vi "exnSpectralBlock spectral measurements peak array WFM.vi"(0 "Signals":waveform(dbl)[](graph), 5 "Restart Averaging":bool, 7 "View":T2, 9 "Spectrum Window":u16, 11 "error in (no error)":errorcluster, 12 "Spectrum Averaging Parameters":T1={"averaging mode"=0, "weighting mode"=1, "number of averages"=10} {"averaging mode" items=["No averaging", "Vector averaging", "RMS averaging", "Peak hold"]; "weighting mode" items=["Linear", "Exponential"]}, 14 "All Spectra":bool) -> (4 "Measurement Output":cluster{"f0":dbl, "df":dbl, "magnitude":dbl[]}[](graph), 6 "averaging done":bool, 10 "Phase":cluster{"f0":dbl, "df":dbl, "phase":dbl[]}[](graph), 15 "error out":errorcluster)   [LabVIEW 2020]
uses:
  <vilib>/measure/NI_MAPro.lvlib
panel:
  in  "measurement":string="FFT - (Peak)"
  in  "string":string=" Phase"
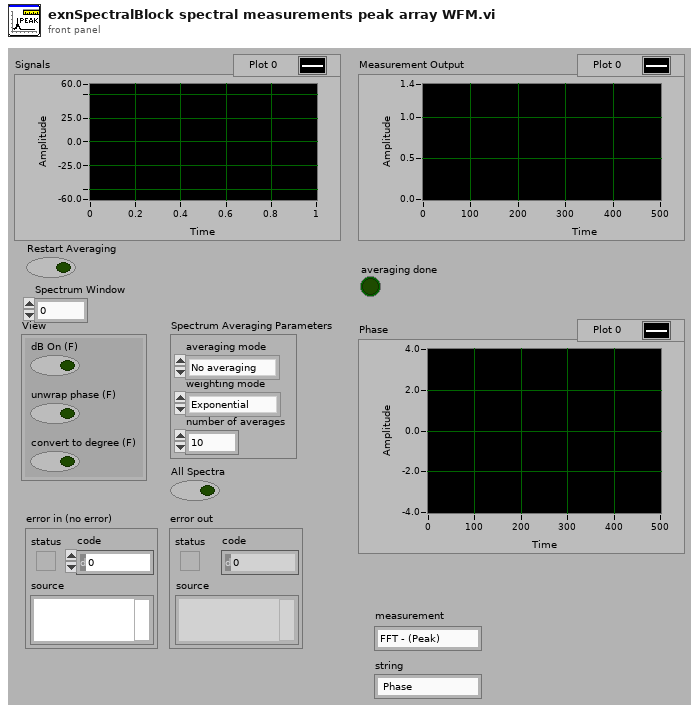
[diagram p1: front panel]
types:
  T1 = cluster{"averaging mode":u16, "weighting mode":u16, "number of averages":u32}
  T2 = cluster{"dB On (F)":bool, "unwrap phase (F)":bool, "convert to degree (F)":bool}
  T3 = enum16{"None ", "Hanning", "Hamming", "Blackman-Harris", "Exact Blackman", "Blackman", "Flat Top", "4 Term B-Harris ", "7 Term B-Harris", "Low Sidelobe"}
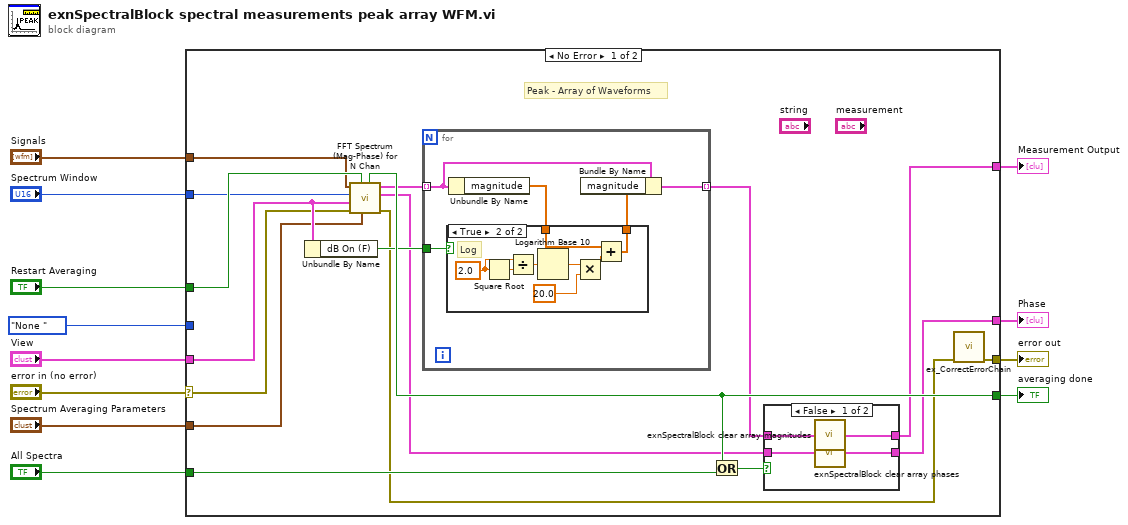
[diagram p0: block diagram]
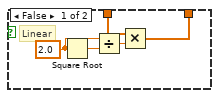
[diagram p2: hidden frame]
diagram:
  n1 = case shown="No Error" "error in (no error)" {
    selector: "error in (no error)" -> [w21 w54]
    tunnel: [w15 _] -> w12
    tunnel: [w14 _] -> w11
    tunnel: [w29 _] -> w10
    tunnel: "All Spectra" -> [w28 _]
    tunnel: "Spectrum Averaging Parameters" -> [w18 _]
    tunnel: "Restart Averaging" -> [w27 _]
    tunnel: T3."None " ("window") -> [_ _]
    tunnel: "Spectrum Window" -> [w22 _]
    tunnel: "View" -> [w26 _]
    tunnel: "Signals" -> [w17 _]
    tunnel: [w25 w54] -> w4
    frame No Error {
      # "Peak - Array of Waveforms"
      n2 = Unbundle By Name(w26) -> ("dB On (F)"=w19:bool)
      n3 = call <vilib>:"FFT Spectrum (Mag-Phase) for N Chan.vi"("averaging parameters"=w18, "restart averaging (F)"=w27, "error in (no error)"=w21, "view"=w26, "window"=w22, "time signals"=w17) -> ("error out"=w16:errorcluster, "phases"=w13:cluster{"f0":dbl, "df":dbl, "phase":dbl[]}[], "magnitudes"=w20:cluster{"f0":dbl, "df":dbl, "magnitude":dbl[]}[], "averaging done"=w29:bool)  [unwired: 1 in, 1 out]
      n4 = for {
        tunnel: [w31] -> w23 mode=indexing
        tunnel: w20 -> [w30] mode=indexing
        tunnel: w19 -> [w33]
        n5 = Unbundle By Name(w30) -> ("magnitude"=w34:dbl[])
        n6 = case shown="True" w33 {
          tunnel: w34 -> [w38 w47]
          tunnel: [w37 w46] -> w32
          frame False {
            w36 = 2.0 ("y")
            # "Linear"
            n7 = Square Root(x=w36) -> (sqrt(x)=w39:dbl)
            n8 = Divide(x=w36, y=w39) -> (x/y=w35:dbl)
            n9 = Multiply(x=w38, y=w35) -> (x*y=w37:dbl[])
          }
          frame True {
            w44 = 2.0 ("y")
            # "Log"
            n10 = Square Root(x=w44) -> (sqrt(x)=w45:dbl)
            n11 = Divide(x=w44, y=w45) -> (x/y=w42:dbl)
            n12 = Logarithm Base 10(1:w42) -> (0:w40:dbl)
            n13 = Multiply(x=w40, y=20.0) -> (x*y=w41:dbl)
            n14 = Add(x=w47, y=w41) -> (x+y=w46:dbl[])
          }
        }
        n15 = Bundle By Name(cluster=w30, "magnitude"=w32) -> (w31:cluster{"f0":dbl, "df":dbl, "magnitude":dbl[]})
      }
      n16 = Or(x=w29, y=w28) -> (x .or. y?=w24:bool)
      n17 = case shown="False" w24 {
        tunnel: w13 -> [w50 w52]
        tunnel: w23 -> [w51 w53]
        tunnel: [w49 w53] -> w15
        tunnel: [w48 w52] -> w14
        frame False {
          n18 = call <vilib>:"exnSpectralBlock clear array magnitudes.vi"("magnitudes in"=w51) -> ("magnitudes out"=w49:cluster{"f0":dbl, "df":dbl, "magnitude":dbl[]}[])
          n19 = call <vilib>:"exnSpectralBlock clear array phases.vi"("phases in"=w50) -> ("phases out"=w48:cluster{"f0":dbl, "df":dbl, "phase":dbl[]}[])
        }
        frame True {
        }
      }
      n20 = call <vilib>:"ex_CorrectErrorChain.vi"("error in (no error)"=w16) -> ("error out"=w25:errorcluster)  [unwired: 10 in]
    }
    frame Error {
    }
  }
  "Phase" <- w11
  "Measurement Output" <- w12
  "averaging done" <- w10
  "error out" <- w4
